vi "ABB Make Sep loss graph.vi"(10 "Show fit":bool, 11 "Results":dbl[][](array[numeric])) -> (1 "Sep Loss Graph":cluster{dbl[], dbl[]}[](graph), 2 "Max Y":dbl, 3 "Rated V Readings":T1)   [LabVIEW 2017]
uses:
  <vilib>/Analysis/NI_AALPro.lvlib
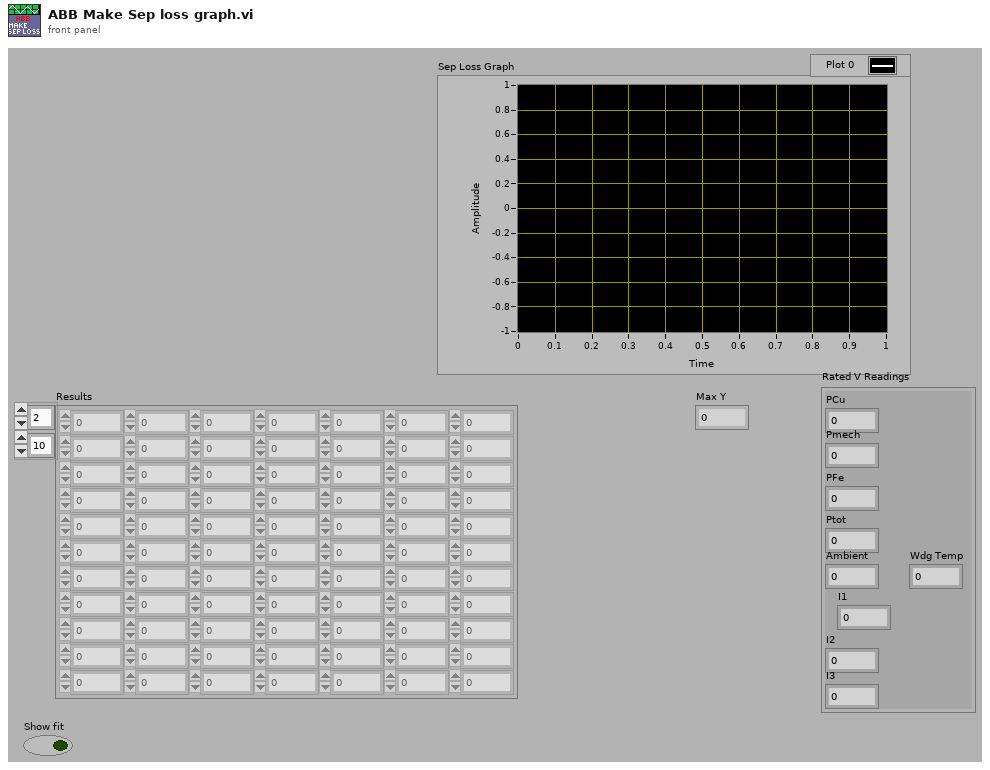
[diagram p1: front panel]
types:
  T1 = cluster{"PCu":dbl, "Pmech":dbl, "PFe":dbl, "Ptot":dbl, "Ambient":dbl, "I1":dbl, "I2":dbl, "I3":dbl, "Wdg Temp":dbl}
  T2 = cluster{"Sorted 2D Array":dbl[], "Best Polynomial Fit":dbl[]}
  T3 = cluster{"Sorted 2D Array":dbl[], "Best Polynomial Fit":dbl[]}[]
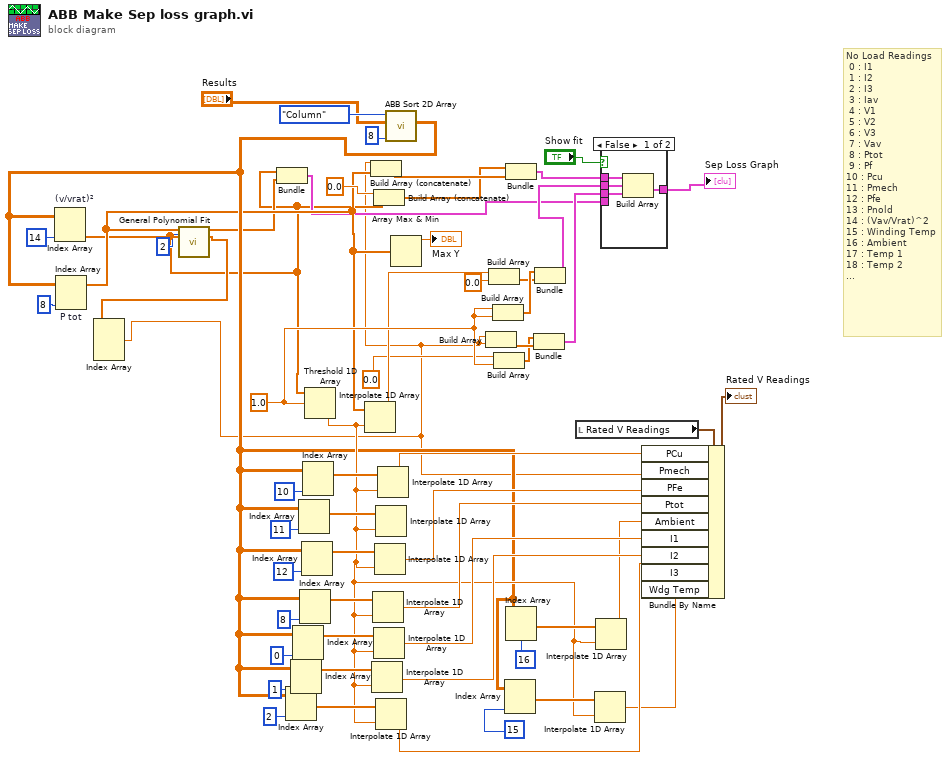
[diagram p0: block diagram]
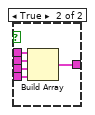
[diagram p2: hidden frame]
diagram:
  w52 = 1.0 ("threshold y")
  # "No Load Readings\n 0 : I1\n 1 : I2\n 2 : I3\n 3 : Iav\n 4 : V1\n 5 : V2\n 6 : V3\n 7 : Vav\n 8 : Ptot\n 9 : Pf\n10 : Pcu\n11 : Pmech\n12 : Pfe\n13 : Pnold\n14 : (Vav/Vrat)^2\n15 : Winding Temp\n16 : Ambient\n17 : Temp 1\n18 : Temp 2\n..."
  n1 = call "ABB Sort 2D Array.vi"("Column/Row to Sort By"=u32 8, "Unsorted 2D Array"="Results", "Sort by"=enum16{"Column", "Row"}."Column") -> ("Sorted 2D Array"=w9:dbl[][])  [unwired: 4 in]
  n2 = Index Array "(v/vrat)²"(array=w9, index (col)=14 ("disabled index (col)")) -> (element=w2:dbl[])  [unwired: 1 in]
  n3 = Index Array "P tot"(array=w9, index (col)=8 ("disabled index (col)")) -> (element=w8:dbl[])  [unwired: 1 in]
  n4 = call <vilib>:"General Polynomial Fit.vi"("Y"=w8, "polynomial order"=2, "X"=w2) -> ("Best Polynomial Fit"=w5:dbl[], "Polynomial Coefficients"=w3:dbl[])  [unwired: 9 in, 2 out]
  n5 = Index Array(array=w3) -> (element #1=w1:dbl)  [unwired: 3 in, 2 out]
  n6 = Bundle("Sorted 2D Array"=w2, "Best Polynomial Fit"=w5) -> (w7:T2)  [unwired: 1 in]
  n7 = Index Array(array=w9, index (col)=2 ("disabled index (col)")) -> (element=w22:dbl[])  [unwired: 1 in]
  n8 = Index Array(array=w9, index (col)=1 ("disabled index (col)")) -> (element=w25:dbl[])  [unwired: 1 in]
  n9 = Index Array(array=w9, index (col)=0 ("disabled index (col)")) -> (element=w26:dbl[])  [unwired: 1 in]
  n10 = Index Array(array=w9, index (col)=11 ("disabled index (col)")) -> (element=w37:dbl[])  [unwired: 1 in]
  n11 = Index Array(array=w9, index (col)=8 ("disabled index (col)")) -> (element=w32:dbl[])  [unwired: 1 in]
  n12 = Index Array(array=w9, index (col)=12 ("disabled index (col)")) -> (element=w36:dbl[])  [unwired: 1 in]
  n13 = Index Array(array=w9, index (col)=10 ("disabled index (col)")) -> (element=w40:dbl[])  [unwired: 1 in]
  n14 = Threshold 1D Array(2:w52, 3:w2) -> (0:w14:dbl)  [unwired: 1 in]
  n15 = Interpolate 1D Array(1:w14, 2:w8) -> (0:w51:dbl)
  n16 = Build Array (concatenate)(w1, w8) -> (w58:dbl[])
  n17 = Interpolate 1D Array(1:w14, 2:w25) -> (0:w20:dbl)
  n18 = Interpolate 1D Array(1:w14, 2:w32) -> (0:w30:dbl)
  n19 = Build Array (concatenate)(0.0, w2) -> (w42:dbl[])
  n20 = Interpolate 1D Array(1:w14, 2:w26) -> (0:w21:dbl)
  n21 = Interpolate 1D Array(1:w14, 2:w36) -> (0:w33:dbl)
  n22 = Interpolate 1D Array(1:w14, 2:w37) -> ()  [unwired: 1 out]
  n23 = Interpolate 1D Array(1:w14, 2:w22) -> (0:w19:dbl)
  n24 = Interpolate 1D Array(1:w14, 2:w40) -> (0:w34:dbl)
  n25 = Array Max & Min(array=w8) -> (max value=→"Max Y":dbl)  [unwired: 3 out]
  n26 = Build Array(w1, w1) -> (w45:dbl[])
  n27 = Build Array(w51, 0.0) -> (w47:dbl[])
  n28 = Build Array(w52, w52) -> (w48:dbl[])
  n29 = Build Array(0.0, w52) -> (w44:dbl[])
  n30 = Index Array(array=w9, index (col)=15 ("disabled index (col)")) -> (element=w15:dbl[])  [unwired: 1 in]
  n31 = Bundle(w42, w58) -> (w50:cluster{dbl[], dbl[]})  [unwired: 1 in]
  n32 = Index Array(array=w9, index (col)=16 ("disabled index (col)")) -> (element=w18:dbl[])  [unwired: 1 in]
  n33 = Bundle(w44, w45) -> (w54:cluster{dbl[], dbl[]})  [unwired: 1 in]
  n34 = Bundle(w48, w47) -> (w53:cluster{dbl[], dbl[]})  [unwired: 1 in]
  n35 = local read "Rated V Readings"() -> (w35:T1)
  n36 = Interpolate 1D Array(1:w14, 2:w15) -> (0:w12:dbl)
  n37 = Interpolate 1D Array(1:w14, 2:w18) -> (0:w16:dbl)
  n38 = case shown="False" "Show fit" {
    tunnel: [w60 w68] -> w59
    tunnel: w54 -> [w61 w67]
    tunnel: w53 -> [w62 w66]
    tunnel: w50 -> [w63 w65]
    tunnel: w7 -> [_ w64]
    frame False {
      n39 = Build Array(w63, w62, w61) -> (w60:cluster{dbl[], dbl[]}[])
    }
    frame True {
      n40 = Build Array(w65, w66, w67, w64) -> (w68:T3)
    }
  }
  "Sep Loss Graph" <- w59
  n41 = Bundle By Name(cluster=w35, "PCu"=w34, "Pmech"=w1, "PFe"=w33, "Ptot"=w30, "Ambient"=w16, "I1"=w21, "I2"=w20, "I3"=w19, "Wdg Temp"=w12) -> (→"Rated V Readings":T1)
